vi "MGI RWA Build Line.vi"(6 "Value String (\"\")":string, 8 "Name In":string, 9 "Array":u32[](array[numeric]), 10 "Iteration":i32, 11 "Iterations":i32) -> (0 "Line":string, 1 "Name Out":string)   [LabVIEW 2016]
doc: "This VI was created for use with the Read/Write Anything VIs. It builds the key name and value line for the INI file for arrays.\n\nAuthored by Robert C. Mortensen\nsupport@mooregoodideas.com\nwww.mooregoodideas.com\n\nCopyright (c) 2010, Moore Good Ideas, Inc.\n\nAll rights reserved.\n\nRedistribution and use in source and binary forms, with or without modification, are permitted provided that the following conditions are met:\n\n * Redistributions of source code must retain the above copyright notice, this list of conditions and the following disclaimer.\n * Redistributions in binary form must reproduce the above copyright notice, this list of conditions and the following disclaimer in the documentation and/or other materials provided with the distribution.\n * Neither the name of Moore Good Ideas, Inc. nor the names of its contributors may be used to endorse or promote products derived from this software without specific prior written permission.\n\nTHIS SOFTWARE IS PROVIDED BY THE COPYRIGHT HOLDERS AND CONTRIBUTORS \"AS IS\" AND ANY EXPRESS OR IMPLIED WARRANTIES, INCLUDING, BUT NOT LIMITED TO, THE IMPLIED WARRANTIES OF MERCHANTABILITY AND FITNESS FOR A PARTICULAR PURPOSE ARE DISCLAIMED. IN NO EVENT SHALL THE COPYRIGHT OWNER OR CONTRIBUTORS BE LIABLE FOR ANY DIRECT, INDIRECT, INCIDENTAL, SPECIAL, EXEMPLARY, OR CONSEQUENTIAL DAMAGES (INCLUDING, BUT NOT LIMITED TO, PROCUREMENT OF SUBSTITUTE GOODS OR SERVICES; LOSS OF USE, DATA, OR PROFITS; OR BUSINESS INTERRUPTION) HOWEVER CAUSED AND ON ANY THEORY OF LIABILITY, WHETHER IN CONTRACT, STRICT LIABILITY, OR TORT (INCLUDING NEGLIGENCE OR OTHERWISE) ARISING IN ANY WAY OUT OF THE USE OF THIS SOFTWARE, EVEN IF ADVISED OF THE POSSIBILITY OF SUCH DAMAGE."
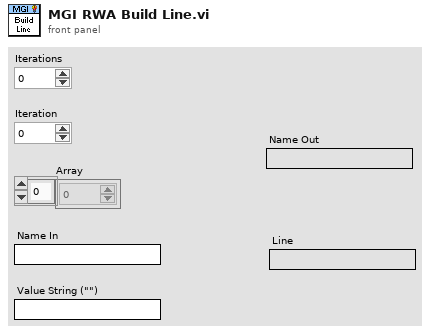
[diagram p1: front panel]
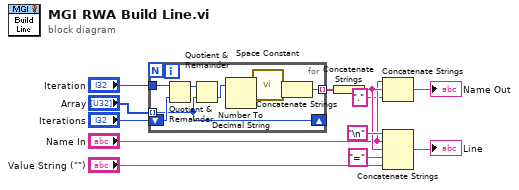
[diagram p0: block diagram]
diagram:
  n1 = for {
    tunnel: [w19] -> w9 mode=indexing
    tunnel: "Iteration" -> [w16]
    tunnel: "Array" -> [w13] mode=indexing
    shift-right: [w13] -> _
    shift-left: "Iterations" -> [w15]
    n2 = Quotient & Remainder(x=w16, y=w15) -> (x-y*floor(x/y)=w17:u32)  [unwired: 1 out]
    n3 = Quotient & Remainder(x=w17, y=w13) -> (floor(x/y)=w14:u32)  [unwired: 1 out]
    n4 = Number To Decimal String(number=w14) -> (decimal integer string=w20:string)  [unwired: 1 in]
    n5 = call <vilib>:"Space Constant.vi"() -> ("String"=w18:string)
    n6 = Concatenate Strings(w18, w20) -> (w19:string)
  }
  n7 = Concatenate Strings(w9) -> (w3:string)
  n8 = Concatenate Strings("Name In", w3, "." ("string")) -> (→"Name Out":string)
  n9 = Concatenate Strings("\n", "Name In", w3, "=" ("string"), "Value String (\"\")") -> (→"Line":string)
